vi "Newmark-SetSpeed.vi"(0 "Table VRN":refnum<visa-resource-name>="COM9", 2 "StageTAG":string, 7 "Bool Refnum":refnum<vi>, 11 "Error IN":errorcluster, 12 "Vitesse Lente":dbl, 13 "Vitesse Rapide":dbl, 14 "Accélération":dbl) -> (4 "Table VRN OUT":refnum<visa-resource-name>="COM9", 8 "Erreur?":bool, 15 "Error OUT":errorcluster)   [LabVIEW 2019]
uses:
  Comm/SerialCommError.vi
panel:
  # "[mm/sec]"
  # "[mm/sec]"
  # "[mm/sec/sec]"
  # "Il faudra probablement vérifier l'ordre dans lequel envoyer les\nvitesse pour respecter l'ordre croissant :\n\nFast en premier, mais si fast en plus petit que la vitesse actuellement\nminimale, on a un problème et on recevra un '#'\n\nNormalement, cela a été réglé ..."
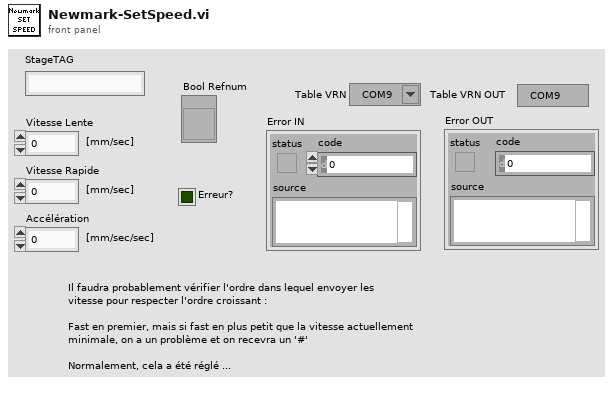
[diagram p1: front panel]
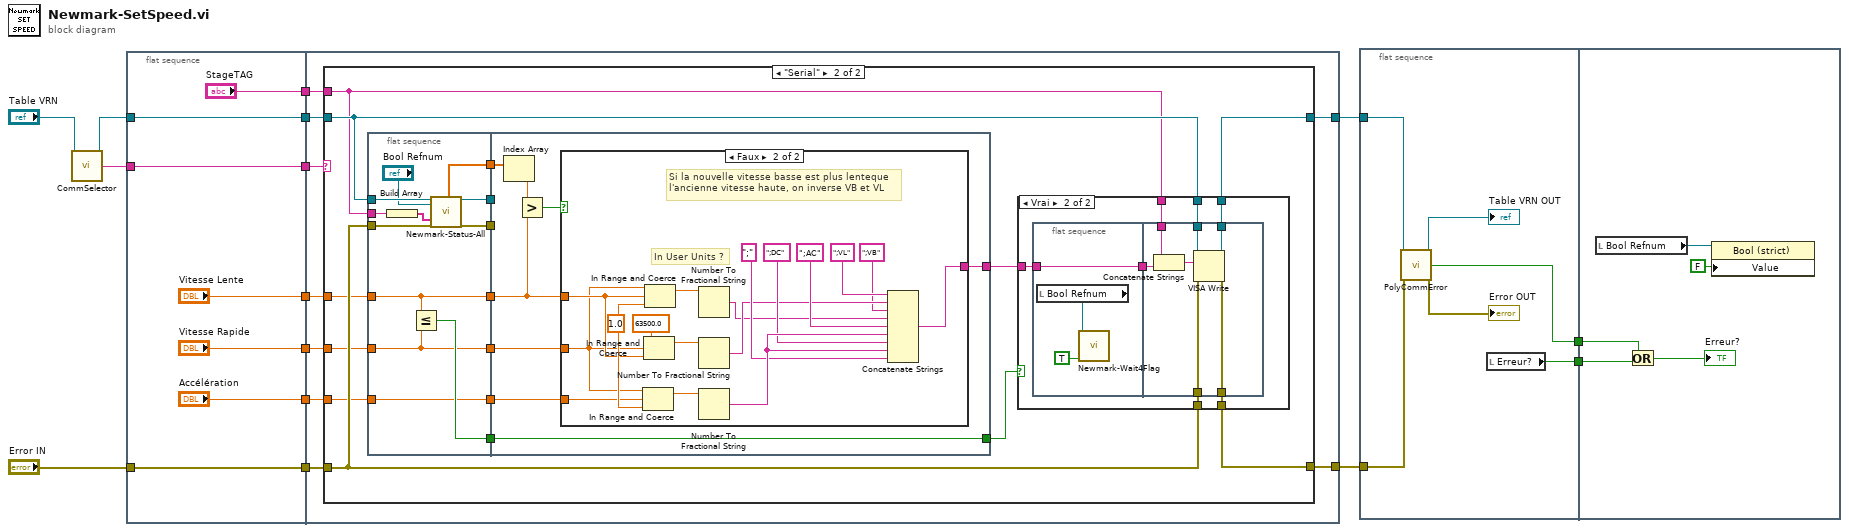
[diagram p0: block diagram]
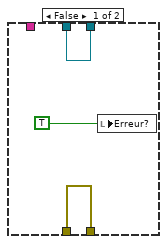
[diagram p3: hidden frame]
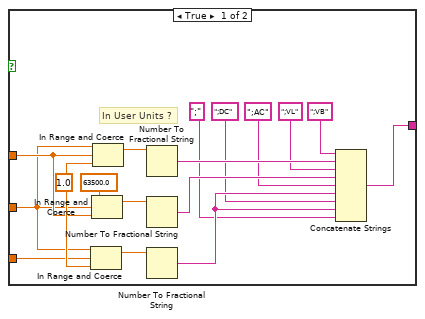
[diagram p4: hidden frame]
diagram:
  n1 = call "CommSelector.vi"("VISA resource name"="Table VRN") -> ("VISA resource name"=w10:refnum<visa-resource-name>, "CommType"=w12:string)  [unwired: 13 in]
  n2 = flat-sequence {
    tunnel: w12 -> [w20]
    tunnel: "Error IN" -> [w21]
    tunnel: w10 -> [w22]
    tunnel: [w22] -> w9
    tunnel: [w21] -> w8
    tunnel: [w20] -> w7
    tunnel: ["Vitesse Lente"] -> w6
    tunnel: ["Vitesse Rapide"] -> w5
    tunnel: ["Accélération"] -> w4
    tunnel: ["StageTAG"] -> w1
    tunnel: [w29] -> w14
    tunnel: [w28] -> w13
    tunnel: w9 -> [w31]
    tunnel: w8 -> [w30]
    tunnel: w7 -> [w27]
    tunnel: w6 -> [w26]
    tunnel: w5 -> [w25]
    tunnel: w4 -> [w24]
    tunnel: w1 -> [w23]
    frame #0 {
    }
    frame #1 {
      n3 = case shown="\"Serial\"" w27 {
        tunnel: w31 -> [w33 w48]
        tunnel: w30 -> [w32 w47]
        tunnel: [w32 w50] -> w29
        tunnel: [w33 w49] -> w28
        tunnel: w26 -> [_ w42]
        tunnel: w25 -> [_ w43]
        tunnel: w24 -> [_ w35]
        tunnel: w23 -> [_ w38]
        frame "Unknown", Default {
        }
        frame "Serial" {
          n4 = flat-sequence {
            tunnel: w48 -> [w82]
            tunnel: w47 -> [w81]
            tunnel: [w79] -> w46
            tunnel: [w78] -> w45
            tunnel: w43 -> [w72]
            tunnel: w42 -> [w76]
            tunnel: [w77] -> w41
            tunnel: [w76] -> w39
            tunnel: w38 -> [w75]
            tunnel: [w73] -> w37
            tunnel: [w72] -> w36
            tunnel: w35 -> [w71]
            tunnel: [w71] -> w34
            tunnel: w46 -> [_]
            tunnel: w45 -> [_]
            tunnel: [w90] -> w44
            tunnel: w41 -> [w89]
            tunnel: [w89] -> w40
            tunnel: w39 -> [w85]
            tunnel: w37 -> [w88]
            tunnel: w36 -> [w84]
            tunnel: w34 -> [w83]
            frame #0 {
              n5 = Build Array(w75) -> (w74:string[])
              n6 = Less Or Equal?(x=w76, y=w72) -> (x <= y?=w77:bool)
              n7 = call "Newmark-Status-All.vi"("Table VRN IN"=w82, "Bool Refnum"="Bool Refnum", "StageTag"=w74, "Error IN"=w81) -> ("?VL"=w73:dbl[], "Table VRN OUT"=w79:refnum<visa-resource-name>, "Error OUT"=w78:errorcluster)  [unwired: 3 in, 10 out]
            }
            frame #1 {
              n8 = Index Array(array=w88) -> (element=w87:dbl)  [unwired: 1 in]
              n9 = Greater?(x=w87, y=w85) -> (0:w86:bool)
              n10 = case shown="Faux" w86 {
                tunnel: [w107 w124] -> w90
                tunnel: w85 -> [w93 w114]
                tunnel: w84 -> [w92 w113]
                tunnel: w83 -> [w91 w112]
                frame True {
                  w99 = 1.0 ("x")
                  # "In User Units ?"
                  n11 = In Range and Coerce(upper limit=w92, x=w91, lower limit=w99) -> (coerced(x)=w101:dbl)  [unwired: 1 out]
                  n12 = In Range and Coerce(upper limit=63500.0 ("x"), x=w92, lower limit=w93) -> (coerced(x)=w102:dbl)  [unwired: 1 out]
                  n13 = In Range and Coerce(upper limit=w92, x=w93, lower limit=w99) -> (coerced(x)=w103:dbl)  [unwired: 1 out]
                  n14 = Number To Fractional String(number=w103) -> (F-format string=w106:string)  [unwired: 3 in]
                  n15 = Number To Fractional String(number=w102) -> (F-format string=w105:string)  [unwired: 3 in]
                  n16 = Number To Fractional String(number=w101) -> (F-format string=w104:string)  [unwired: 3 in]
                  n17 = Concatenate Strings(";VB" ("string"), w106, ";VL" ("string"), w105, ";AC" ("string"), w104, ";DC" ("string"), w104, ";" ("string")) -> (w107:string)
                }
                frame False {
                  w118 = 1.0 ("x")
                  # "Si la nouvelle vitesse basse est plus lenteque\nl'ancienne vitesse haute, on inverse VB et VL"
                  # "In User Units ?"
                  n18 = In Range and Coerce(upper limit=w113, x=w112, lower limit=w118) -> (coerced(x)=w120:dbl)  [unwired: 1 out]
                  n19 = In Range and Coerce(upper limit=63500.0 ("x"), x=w113, lower limit=w114) -> (coerced(x)=w121:dbl)  [unwired: 1 out]
                  n20 = In Range and Coerce(upper limit=w113, x=w114, lower limit=w118) -> (coerced(x)=w122:dbl)  [unwired: 1 out]
                  n21 = Number To Fractional String(number=w122) -> (F-format string=w109:string)  [unwired: 3 in]
                  n22 = Number To Fractional String(number=w121) -> (F-format string=w110:string)  [unwired: 3 in]
                  n23 = Number To Fractional String(number=w120) -> (F-format string=w123:string)  [unwired: 3 in]
                  n24 = Concatenate Strings(";VL" ("string"), w110, ";VB" ("string"), w109, ";AC" ("string"), w123, ";DC" ("string"), w123, ";" ("string")) -> (w124:string)
                }
              }
            }
          }
          n25 = case shown="Vrai" w40 {
            tunnel: [w52 w59] -> w50
            tunnel: [w53 w58] -> w49
            tunnel: w48 -> [w53 w57]
            tunnel: w47 -> [w52 w56]
            tunnel: w38 -> [_ w55]
            tunnel: w44 -> [_ w54]
            frame False {
              n26 = local write "Erreur?"(TRUE ("Erreur?")) -> ()
            }
            frame True {
              n27 = flat-sequence {
                tunnel: w54 -> [w63]
                tunnel: [w63] -> w60
                tunnel: [w70] -> w59
                tunnel: [w69] -> w58
                tunnel: w57 -> [w68]
                tunnel: w56 -> [w67]
                tunnel: w55 -> [w65]
                tunnel: w60 -> [w64]
                frame #0 {
                  n28 = local read "Bool Refnum"() -> (w62:refnum<vi>)
                  n29 = call "Newmark-Wait4Flag.vi"("Raise Flag ?"=TRUE, "Ctl Refnum IN"=w62) -> ()  [unwired: 8 in, 2 out]
                }
                frame #1 {
                  n30 = Concatenate Strings(w65, w64) -> (w66:string)
                  n31 = VISA Write(VISA resource name=w68, write buffer=w66, error in (no error)=w67) -> (VISA resource name out=w69:refnum<visa-resource-name>, error out=w70:errorcluster)  [unwired: 1 out]
                }
              }
            }
          }
        }
      }
    }
  }
  n32 = flat-sequence {
    tunnel: w14 -> [w129]
    tunnel: w13 -> [w130]
    tunnel: [w126] -> w3
    tunnel: [w125] -> w2
    tunnel: w3 -> [w132]
    tunnel: w2 -> [w133]
    frame #0 {
      n33 = call-poly "PolyCommError.vi"("VISA IN"=w130, "error IN"=w129) -> ("VISA OUT"=→"Table VRN OUT":refnum<visa-resource-name>, "Error"=w126:bool, "error OUT"=→"Error OUT":errorcluster)  [unwired: 11 in]
      n34 = local read "Erreur?"() -> (w125:bool)
    }
    frame #1 {
      n35 = local read "Bool Refnum"() -> (w134:refnum<vi>)
      n36 = Or(x=w132, y=w133) -> (x .or. y?=→"Erreur?":bool)
      n37 = property class="Bool (strict)"(reference=w134, "Value"=FALSE) -> ()  [unwired: 1 in, 2 out]
    }
  }
